vi "Read Home Params Cluster.vi"(8 "error in (no error)":errorcluster, 11 "Motor in":refnum<class "Motor.lvclass">) -> (0 "error out":errorcluster, 2 "Home Params Cluster":T1={"Home Mode"=enum."EZ+EL", "Home Dir"=enum."positive+", "Home Pos Shift"=0.0}, 3 "Motor out":refnum<class "Motor.lvclass">)   [LabVIEW 2016, in "Hardware.lvlib" / "Motor.lvlib" / "Motor.lvclass"]
uses:
  <userlib>/Common Components/Hardware/Motor/Motor/Motor.lvclass
  <userlib>/Common Components/Hardware/Motor/Motor/Home Params.ctl
  <userlib>/Common Components/Hardware/Motor/Motor/Home Mode.ctl
  <userlib>/Common Components/Hardware/Motor/Motor/Home Dir.ctl
  <userlib>/Common Components/Hardware/Motor/Motor/Motor.lvclass/Motor.ctl
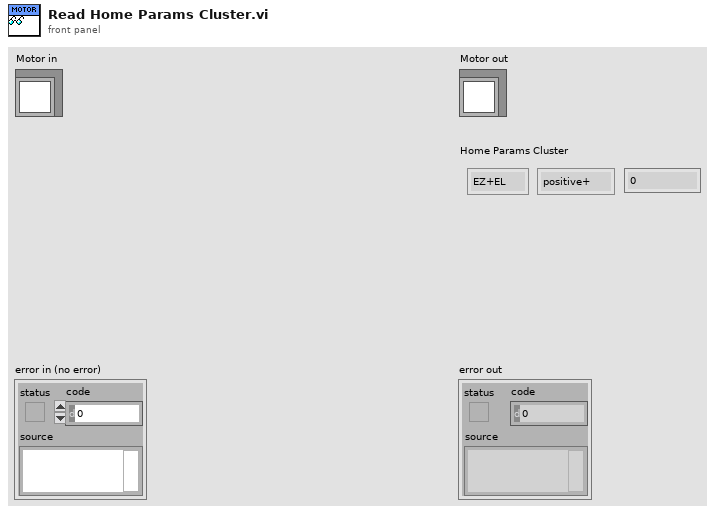
[diagram p1: front panel]
types:
  T1 = typedef "Hardware.lvlib/Motor.lvlib/Motor.lvclass/Home Params.ctl" = cluster{"Home Mode":T2, "Home Dir":T3, "Home Pos Shift":dbl}
  T2 = typedef "Hardware.lvlib/Motor.lvlib/Motor.lvclass/Home Mode.ctl" = enum16{"EZ+EL", "EZ only"}
  T3 = typedef "Hardware.lvlib/Motor.lvlib/Motor.lvclass/Home Dir.ctl" = enum16{"negative-", "positive+"}
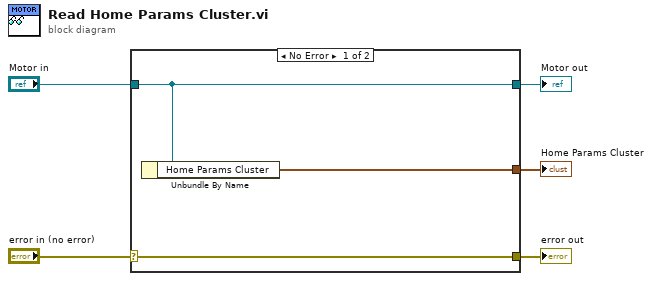
[diagram p0: block diagram]
diagram:
  n1 = case shown="No Error" "error in (no error)" {
    selector: "error in (no error)" -> [w8 w9]
    tunnel: [w8 w9] -> w4
    tunnel: [w7 w10] -> w2
    tunnel: "Motor in" -> [w7 w10]
    tunnel: [w6 _] -> w1
    frame No Error {
      n2 = Unbundle By Name(w7) -> ("Home Params Cluster"=w6:T1)
    }
    frame Error {
    }
  }
  "error out" <- w4
  "Motor out" <- w2
  "Home Params Cluster" <- w1
